vi "ParamsAMgen.vi"(2 "paramsIn":variant) -> (16 "paramsOut":variant)   [LabVIEW 2017]
uses:
  Typedefs/Tipo_ComponenteSinalRuidoComposto.ctl
  Typedefs/Tipo_TipoSinalCarrier.ctl
  Typedefs/Tipo_ParamsAMgen.ctl
panel:
  in  "Tipo":T1
  in  "Ruído Total":dbl
  in  "Modulation":dbl
  in  "Carrier Frequency":dbl
  in  "Componentes":T2[](array[typedef])=[{"Amplit.: "=0.0, "Freq. (Hz): "=0.0, "Fase (º):"=0.0, "Ruido"=0.0}, {"Amplit.: "=0.0, "Freq. (Hz): "=0.0, "Fase (º):"=0.0, "Ruido"=0.0}, {"Amplit.: "=0.0, "Freq. (Hz): "=0.0, "Fase (º):"=0.0, "Ruido"=0.0}, {"Amplit.: "=0.0, "Freq. (Hz): "=0.0, "Fase (º):"=0.0, "Ruido"=0.0}]
  in  "Init":bool
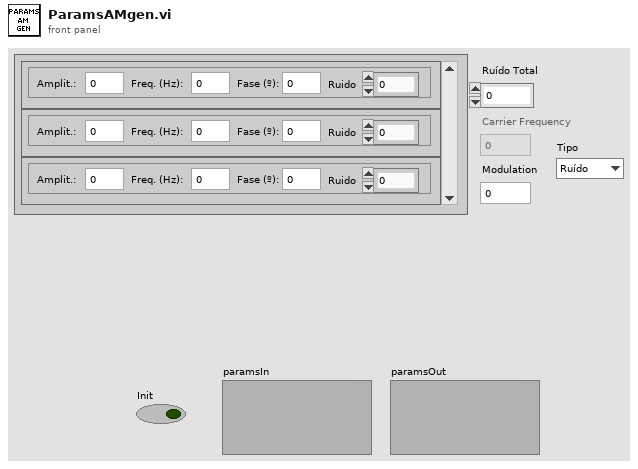
[diagram p1: front panel]
types:
  T1 = typedef "Tipo_TipoSinalCarrier.ctl" = enum16{"Ruído", "Senóide"}
  T2 = typedef "Tipo_ComponenteSinalRuidoComposto.ctl" = cluster{"Amplit.: ":dbl, "Freq. (Hz): ":dbl, "Fase (º):":dbl, "Ruido":dbl}
  T3 = typedef "Tipo_ParamsAMgen.ctl" = cluster{"Componentes":T2[], "Carrier Frequency":dbl, "Modulation":dbl, "Ruído Total":dbl, "Tipo":T1}
  T4 = enum8{"Enabled", "Disabled", "Disabled and Grayed Out"}
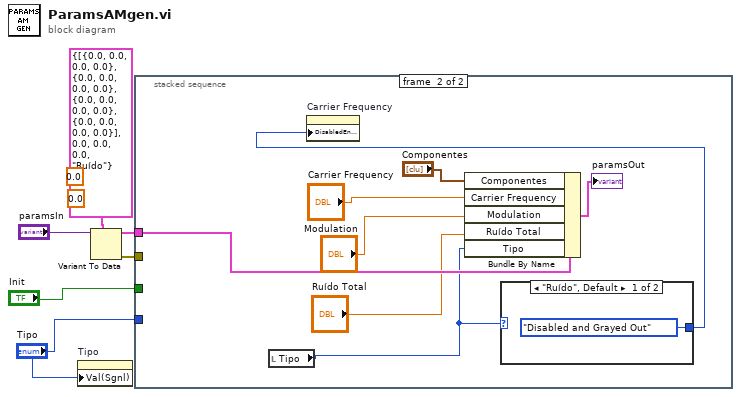
[diagram p0: block diagram]
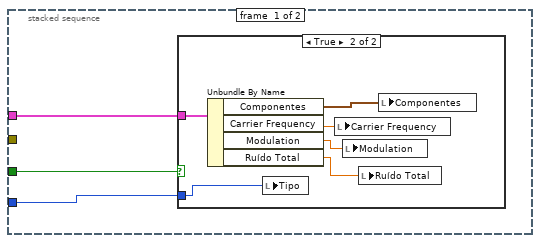
[diagram p2: hidden frame]
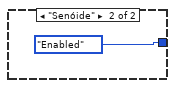
[diagram p4: hidden frame]
diagram:
  (unwired) 0.0 ("Ruído")
  (unwired) 0.0 ("Ruído")
  n1 = property on="Tipo" class="Enum (strict)"("Val(Sgnl)"="Tipo") -> ()  [unwired: 2 in, 2 out]
  n2 = Variant To Data(type=T3 {"Componentes"=[{"Amplit.: "=0.0, "Freq. (Hz): "=0.0, "Fase (º):"=0.0, "Ruido"=0.0}, {"Amplit.: "=0.0, "Freq. (Hz): "=0.0, "Fase (º):"=0.0, "Ruido"=0.0}, {"Amplit.: "=0.0, "Freq. (Hz): "=0.0, "Fase (º):"=0.0, "Ruido"=0.0}, {"Amplit.: "=0.0, "Freq. (Hz): "=0.0, "Fase (º):"=0.0, "Ruido"=0.0}], "Carrier Frequency"=0.0, "Modulation"=0.0, "Ruído Total"=0.0, "Tipo"=enum."Ruído"} ("Cluster"), Variant="paramsIn") -> (data=w5:T3, error out=w3:errorcluster)  [unwired: 1 in]
  n3 = stacked-sequence {
    tunnel: w5 -> [w9 w23]
    tunnel: "Init" -> [w8 _]
    tunnel: w3 -> [_ _]
    tunnel: "Tipo" -> [w7 _]
    frame #0 {
      n4 = case shown="True" w8 {
        tunnel: w9 -> [_ w15]
        tunnel: w7 -> [_ w10]
        frame False {
        }
        frame True {
          n5 = Unbundle By Name(w15) -> ("Componentes"=w14:T2[], "Carrier Frequency"=w13:dbl, "Modulation"=w12:dbl, "Ruído Total"=w11:dbl)
          n6 = local write "Tipo"(w10) -> ()
          n7 = local write "Carrier Frequency"(w13) -> ()
          n8 = local write "Modulation"(w12) -> ()
          n9 = local write "Ruído Total"(w11) -> ()
          n10 = local write "Componentes"(w14) -> ()
        }
      }
    }
    frame #1 {
      n11 = local read "Tipo"() -> (w17:T1)
      n12 = Bundle By Name(cluster=w23, "Componentes"="Componentes", "Carrier Frequency"="Carrier Frequency", "Modulation"="Modulation", "Ruído Total"="Ruído Total", "Tipo"=w17) -> (→"paramsOut":T3)
      n13 = case shown="\"Ruído\", Default" w17 {
        tunnel: [T4."Disabled and Grayed Out" ("Disabled") T4."Enabled" ("Disabled")] -> w16
        frame "Ruído", Default {
        }
        frame "Senóide" {
        }
      }
      n14 = property on="Carrier Frequency" class="DigNum (strict)"("DisabledEnum"=w16) -> ()  [unwired: 2 in, 2 out]
    }
  }
